vi "Read Header from file.vi"(6 "error in":errorcluster, 9 "File":refnum<file>) -> (0 "error out":errorcluster, 1 "ImFileDirectOffs":u32, 2 "Litt/BigEnd":bool, 3 "File":refnum<file>, 4 "isTIFF":bool)   [LabVIEW 2013, in "Tiff reader.lvlib"]
doc: "Reads the header of a tiff file to determine the version number and the location of the image data in the file. Format determines whether the image file is coded LSB or MSB, although the rest of the routines only understand PC image data !"
uses:
  Tiff reader.lvlib
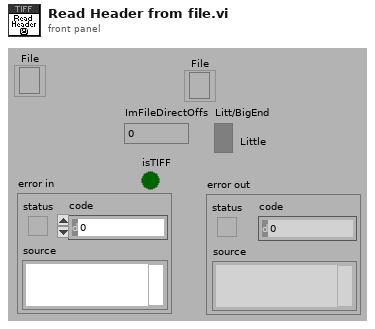
[diagram p1: front panel]
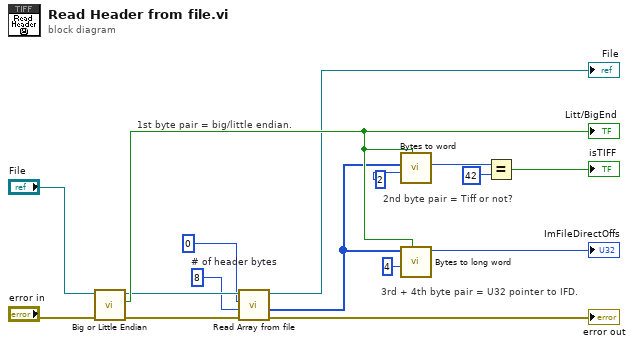
[diagram p0: block diagram]
diagram:
  w4 = 8  # # of header bytes
  # "3rd + 4th byte pair = U32 pointer to IFD."
  # "2nd byte pair = Tiff or not?"
  # "1st byte pair = big/little endian."
  n1 = call "Big or Little Endian.vi"("error in"="error in", "File"="File") -> ("error out"=w6:errorcluster, "Litt/BigEnd"=w8:bool, "File out"=w7:refnum<file>)  [unwired: 7 out]
  "Litt/BigEnd" <- w8
  n2 = call "Read Array from file.vi"("error in"=w6, "bytes to read"=w4, "File location in"=i64 0, "File"=w7) -> ("error out"=→"error out":errorcluster, "Array of U8s"=w2:u8[], "File out"=→"File":refnum<file>)  [unwired: 1 out]
  n3 = call "Bytes to word.vi"("Litt/BigEnd"=w8, "Index"=2, "Image Data in"=w2) -> ("Word"=w12:u16)  [unwired: 1 in, 5 out]
  n4 = call "Bytes to long word.vi"("Litt/BigEnd"=w8, "Index"=4, "Image Data in"=w2) -> ("U32"=→"ImFileDirectOffs":u32)  [unwired: 6 out]
  n5 = Equal?(x=w12, y=u16 42 ("Word")) -> (x = y?=→"isTIFF":bool)
